vi "RunJavaScript.vi"(0 "reference in":refnum<class "LcWebView.lvclass">, 1 "Java Script Function":string="document.documentElement.outerHTML", 5 "Error In":errorcluster) -> (14 "reference out":refnum<class "LcWebView.lvclass">, 15 "Result":string, 16 "Status":i32(ring) items=["Created", "WaitingForActivation", "WaitingToRun", "Running", "WaitingForChildrenToComplete", "RanToCompletion", "Canceled", "Faulted"], 19 "Error Out":errorcluster)   [LabVIEW 2021, in "LcWebView.lvclass"]
doc: "Get HTML comtent"
uses:
  LcWebView.lvclass
  C:/Users/ziggz/OneDrive/Documents/GitHub/LcWebView2/LcWebView/data/Microsoft.Web.WebView2.Core.dll
  data/Microsoft.Web.WebView2.Core.dll
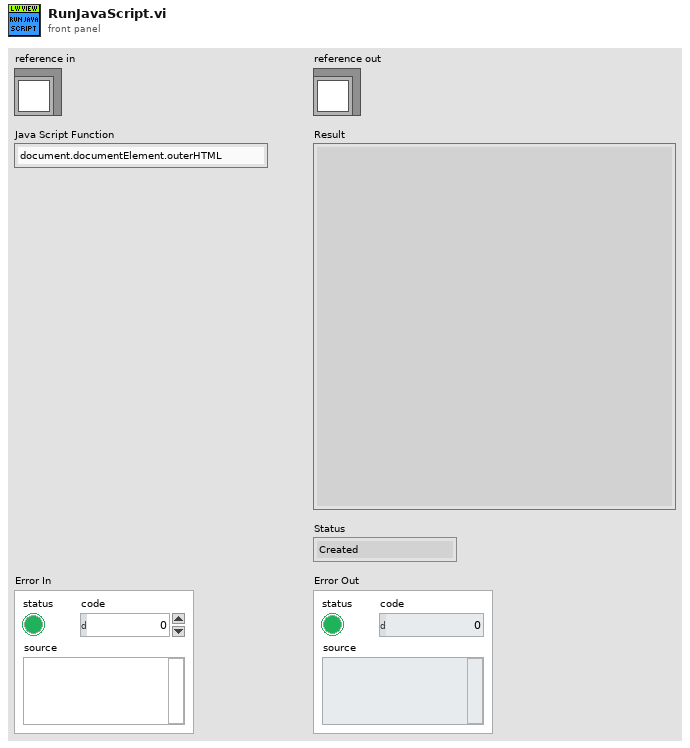
[diagram p1: front panel]
types:
  T1 = typedef "LcWebView.lvclass/ObjectAttributes.ctl" = cluster{"WebView Container":refnum<k24>, "CoreWebViewRef":refnum<k24>, "Status":i32, "Status Message":string, "User Data Folder":path, "BrowserProcessId":u32, "PlotType":T2}
  T2 = typedef "LcWebView.lvclass/PlotType.ctl" = enum16{"bar", "line", "pie", "doughnut", "scatter", "radar", "bubble", "polarArea"}
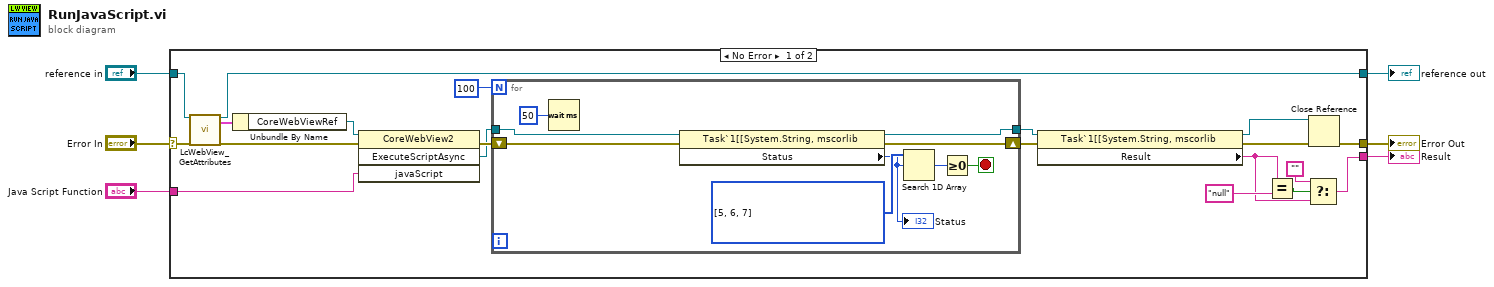
[diagram p0: block diagram]
diagram:
  n1 = case shown="No Error" "Error In" {
    selector: "Error In" -> [w26 w37]
    tunnel: [w12 w37] -> w5
    tunnel: [w23 w36] -> w3
    tunnel: "reference in" -> [w24 w36]
    tunnel: [w7 _] -> w2
    tunnel: "Java Script Function" -> [w15 _]
    frame No Error {
      n2 = call "LcWebView_GetAttributes.vi"("reference in"=w24, "error in (no error)"=w26) -> ("reference out"=w23:refnum<class "LcWebView.lvclass">, "Data"=w25:T1, "error out"=w21:errorcluster)  [unwired: 14 in, 1 out]
      n3 = Unbundle By Name(w25) -> ("CoreWebViewRef"=w22:refnum<k24>)
      n4 = invoke class="CoreWebView2" method="ExecuteScriptAsync"(reference=w22, error in=w21, "javaScript"=w15) -> (error out=w20:errorcluster, "ExecuteScriptAsync"=w16:refnum<k24>)  [unwired: 1 in, 2 out]
      n5 = for {
        N: 100 -> [_]
        tunnel: w16 -> [w35]
        shift-right: [w33] -> w17
        shift-left: w20 -> [w34]
        tunnel: [w31] -> w18
        stop <- w27 stop-if-true
        w30 = i32[] [5, 6, 7] items=["Created", "WaitingForActivation", "WaitingToRun", "Running", "WaitingForChildrenToComplete", "RanToCompletion", "Canceled", "Faulted"] ("Status")
        n6 = Wait (ms)(milliseconds to wait=u32 50) -> ()  [unwired: 1 out]
        n7 = property class="Task`1[[System.String, mscorlib"(reference=w35, error in=w34) -> (reference out=w31:refnum<k24>, error out=w33:errorcluster, "Status"=w29:i32)
        "Status" <- w29
        n8 = Search 1D Array(1D array=w30, element=w29) -> (index of element=w28:i32)  [unwired: 1 in]
        n9 = Greater Or Equal To 0?(x=w28) -> (x >= 0?=w27:bool)
      }
      n10 = property class="Task`1[[System.String, mscorlib"(reference=w18, error in=w17) -> (reference out=w14:refnum<k24>, error out=w13:errorcluster, "Result"=w8:string)
      n11 = Equal?(x=w8, y="null") -> (x = y?=w10:bool)
      n12 = Select(t="", s=w10, f=w8) -> (s? t:f=w7:string)
      n13 = Close Reference(reference=w14, error in (no error)=w13) -> (error out=w12:errorcluster)
    }
    frame Error {
    }
  }
  "Error Out" <- w5
  "reference out" <- w3
  "Result" <- w2
